vi "main.vi"() -> ()   [LabVIEW 2015]
panel:
  in  "Attenuation":string(combo)
  in  "Level":dbl
  in  "Cmos":string(combo)
  in  "Duty":dbl
  in  "Modulation":string(combo)
  in  "Frequency":dbl
  in  "Range":string(combo)
  in  "Offset":dbl
  in  "Counter":string(combo)
  out "error in":errorcluster
  out "error out":errorcluster
  in  "Function type":string(combo)
  in  "close":bool=TRUE
  out "VISA resource name out":refnum<visa-resource-name>
  in  "open":bool=TRUE
  in  "VISA resource name":refnum<visa-resource-name>
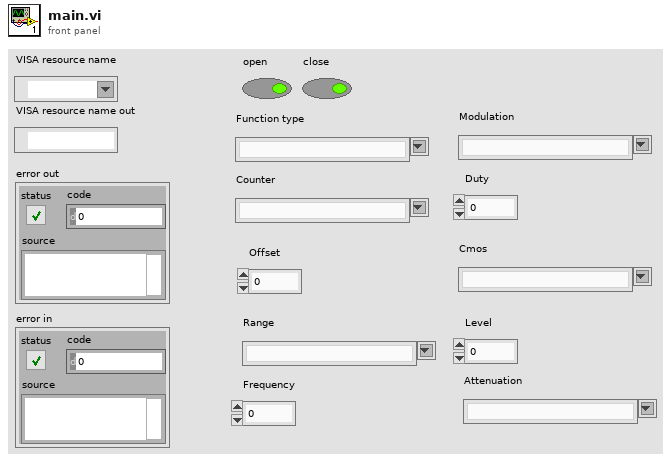
[diagram p1: front panel]
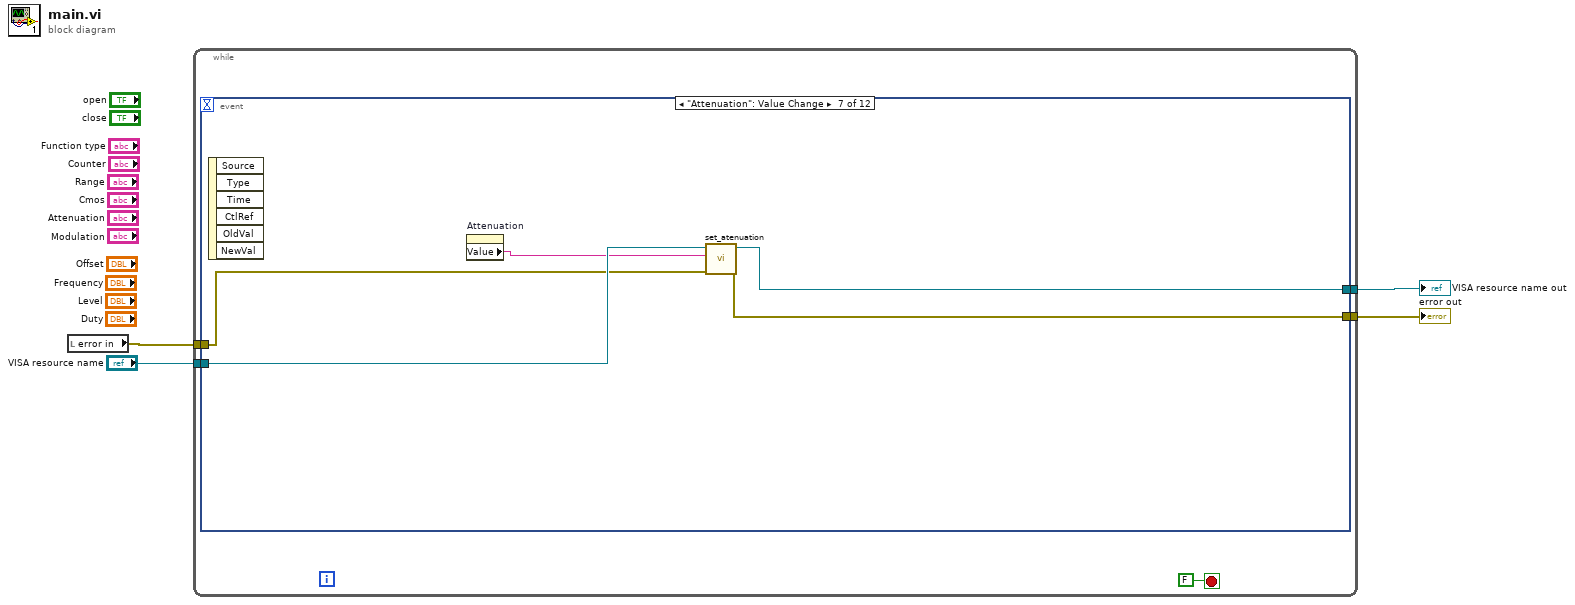
[diagram p0: block diagram]
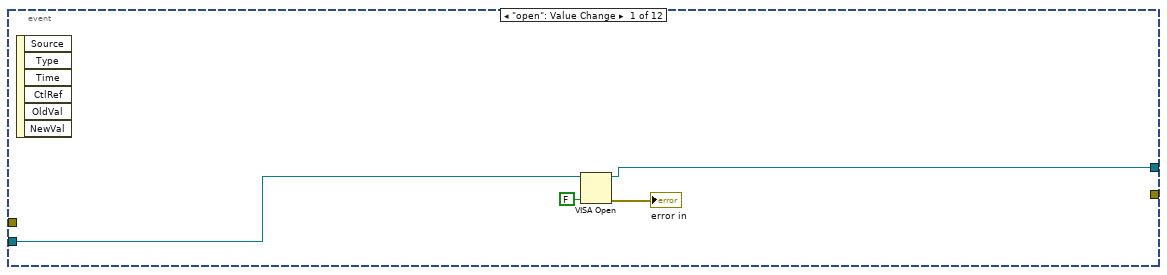
[diagram p2: hidden frame]
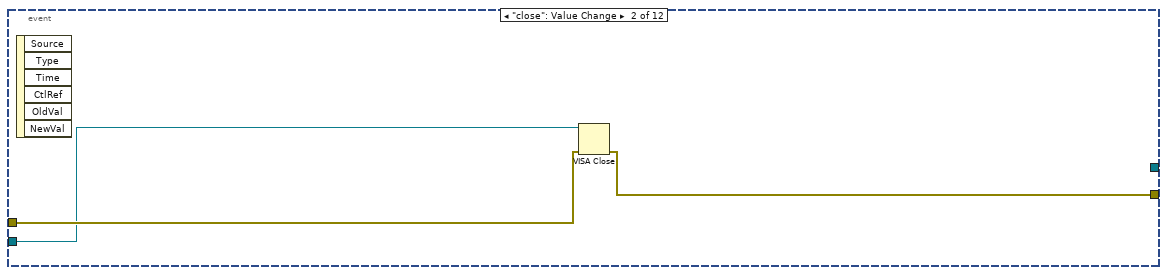
[diagram p3: hidden frame]
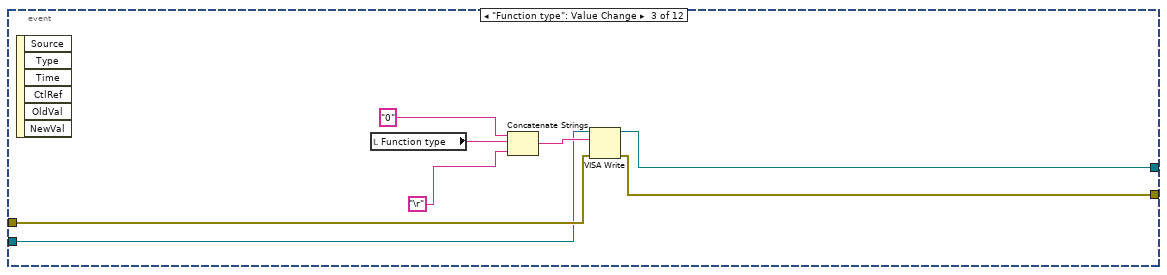
[diagram p4: hidden frame]
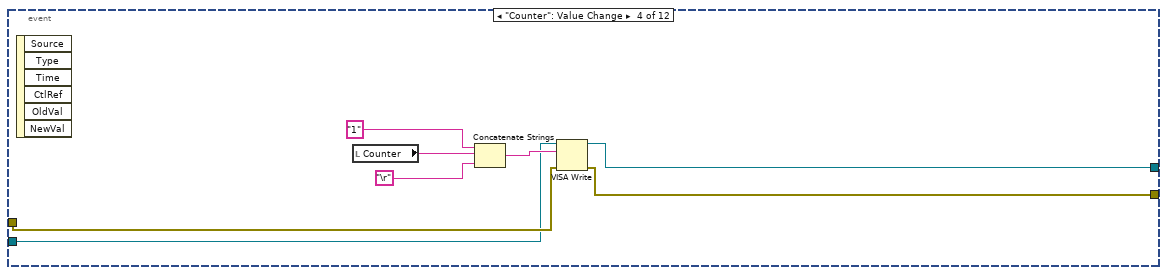
[diagram p5: hidden frame]
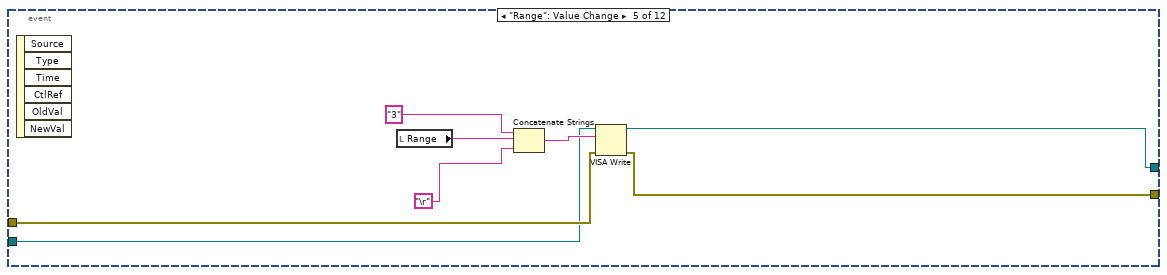
[diagram p6: hidden frame]
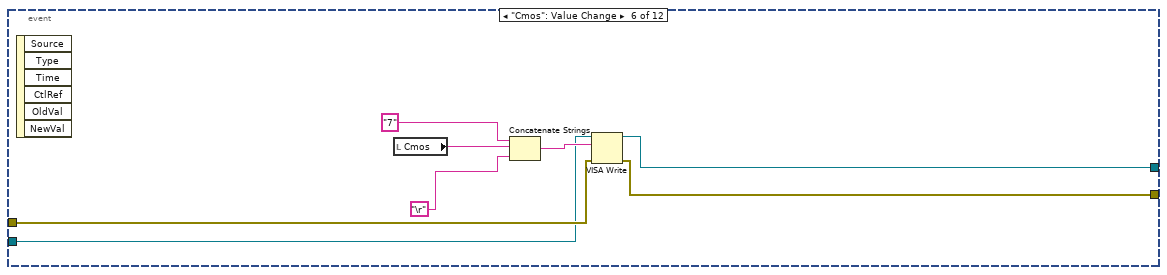
[diagram p7: hidden frame]
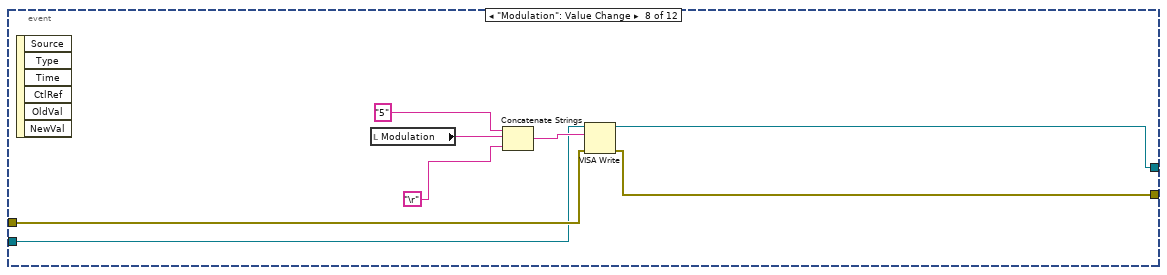
[diagram p8: hidden frame]
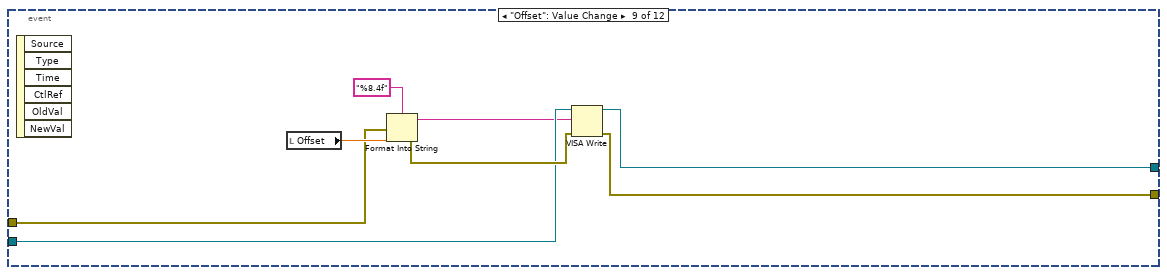
[diagram p9: hidden frame]
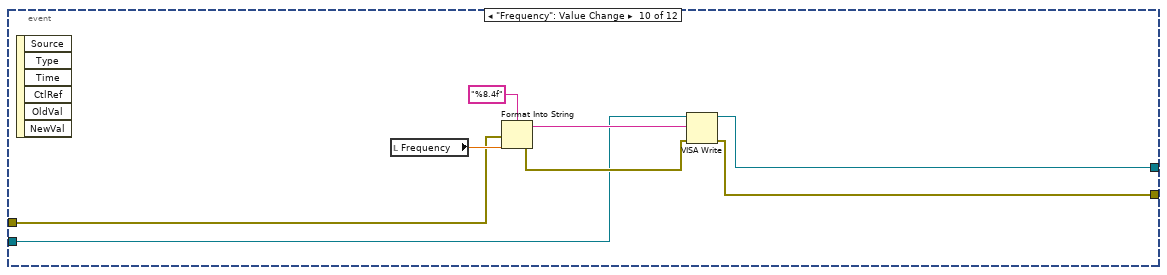
[diagram p10: hidden frame]
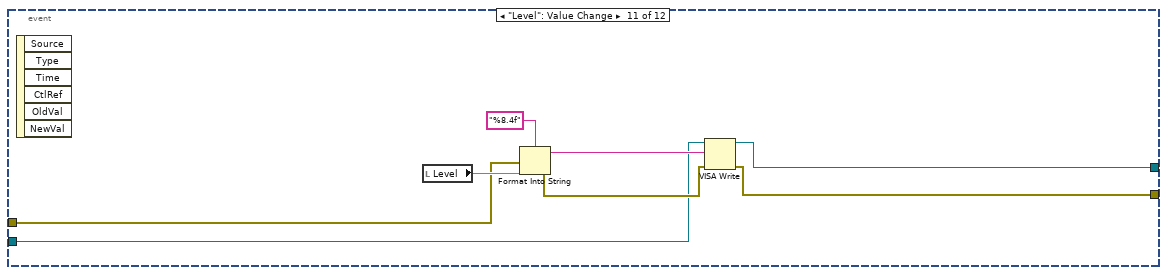
[diagram p11: hidden frame]
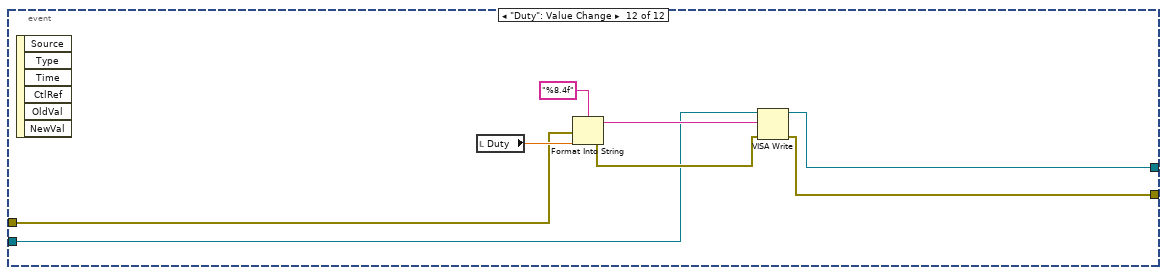
[diagram p12: hidden frame]
diagram:
  n1 = local read "error in"() -> (w4:errorcluster)
  n2 = while {
    tunnel: w4 -> [w8]
    tunnel: [w7] -> w3
    tunnel: "VISA resource name" -> [w6]
    tunnel: [w5] -> w1
    stop <- FALSE ("stop") stop-if-true
    n3 = event shown="[6] \"Attenuation\": Value Change" {
      selector: _ -> [_ _ _ _ _ _ _ _ _ _ _ _]
      dyn-events: _ -> [_ _ _ _ _ _ _ _ _ _ _ _]
      timeout: _ -> [_ _ _ _ _ _ _ _ _ _ _ _]
      tunnel: w8 -> [_ w16 w20 w28 w36 w44 w52 w57 w67 w73 w81 w89]
      tunnel: [_ w15 w19 w27 w33 w42 w50 w54 w65 w70 w79 w86] -> w7
      tunnel: w6 -> [w11 w14 w18 w25 w35 w43 w53 w56 w64 w72 w80 w88]
      tunnel: [w10 _ w17 w26 w34 w41 w51 w55 w62 w71 w78 w87] -> w5
      event "open": Value Change {
        n4 = event-data() -> ()  [unwired: 1 in, 6 out]
        n5 = VISA Open(duplicate session (F)=FALSE, VISA resource name=w11) -> (VISA resource name=w10:refnum<visa-resource-name>, error out=→"error in":errorcluster)  [unwired: 3 in]
      }
      event "close": Value Change {
        n6 = event-data() -> ()  [unwired: 1 in, 6 out]
        n7 = VISA Close(VISA resource name=w14, error in (no error)=w16) -> (error out=w15:errorcluster)
      }
      event "Function type": Value Change {
        n8 = event-data() -> ()  [unwired: 1 in, 6 out]
        n9 = local read "Function type"() -> (w24:string)
        n10 = Concatenate Strings("0" ("string"), w24, "\r") -> (w22:string)
        n11 = VISA Write(VISA resource name=w18, write buffer=w22, error in (no error)=w20) -> (VISA resource name out=w17:refnum<visa-resource-name>, error out=w19:errorcluster)  [unwired: 1 out]
      }
      event "Counter": Value Change {
        n12 = event-data() -> ()  [unwired: 1 in, 6 out]
        n13 = local read "Counter"() -> (w29:string)
        n14 = Concatenate Strings("1" ("string"), w29, "\r") -> (w31:string)
        n15 = VISA Write(VISA resource name=w25, write buffer=w31, error in (no error)=w28) -> (VISA resource name out=w26:refnum<visa-resource-name>, error out=w27:errorcluster)  [unwired: 1 out]
      }
      event "Range": Value Change {
        n16 = event-data() -> ()  [unwired: 1 in, 6 out]
        n17 = local read "Range"() -> (w37:string)
        n18 = Concatenate Strings("3" ("string"), w37, "\r") -> (w39:string)
        n19 = VISA Write(VISA resource name=w35, write buffer=w39, error in (no error)=w36) -> (VISA resource name out=w34:refnum<visa-resource-name>, error out=w33:errorcluster)  [unwired: 1 out]
      }
      event "Cmos": Value Change {
        n20 = event-data() -> ()  [unwired: 1 in, 6 out]
        n21 = local read "Cmos"() -> (w45:string)
        n22 = Concatenate Strings("7" ("string"), w45, "\r") -> (w47:string)
        n23 = VISA Write(VISA resource name=w43, write buffer=w47, error in (no error)=w44) -> (VISA resource name out=w41:refnum<visa-resource-name>, error out=w42:errorcluster)  [unwired: 1 out]
      }
      event "Attenuation": Value Change {
        n24 = event-data() -> ()  [unwired: 1 in, 6 out]
        n25 = property on="Attenuation" class="CmbBox"() -> ("Value"=w49:string)  [unwired: 2 in, 2 out]
        n26 = call "set_atenuation.vi"("error in (no error)"=w52, "Value"=w49, "VISA Refnum in"=w53) -> ("error out"=w50:errorcluster, "VISA Refnum out"=w51:refnum<visa-resource-name>)  [unwired: 7 in]
      }
      event "Modulation": Value Change {
        n27 = event-data() -> ()  [unwired: 1 in, 6 out]
        n28 = local read "Modulation"() -> (w58:string)
        n29 = Concatenate Strings("5" ("string"), w58, "\r") -> (w60:string)
        n30 = VISA Write(VISA resource name=w56, write buffer=w60, error in (no error)=w57) -> (VISA resource name out=w55:refnum<visa-resource-name>, error out=w54:errorcluster)  [unwired: 1 out]
      }
      event "Offset": Value Change {
        n31 = event-data() -> ()  [unwired: 1 in, 6 out]
        n32 = local read "Offset"() -> (w69:dbl)
        n33 = Format Into String(format string="%8.4f", error in=w67, w69) -> (resulting string=w63:string, error out=w66:errorcluster)  [unwired: 1 in]
        n34 = VISA Write(VISA resource name=w64, write buffer=w63, error in (no error)=w66) -> (VISA resource name out=w62:refnum<visa-resource-name>, error out=w65:errorcluster)  [unwired: 1 out]
      }
      event "Frequency": Value Change {
        n35 = event-data() -> ()  [unwired: 1 in, 6 out]
        n36 = local read "Frequency"() -> (w77:dbl)
        n37 = Format Into String(format string="%8.4f", error in=w73, w77) -> (resulting string=w74:string, error out=w75:errorcluster)  [unwired: 1 in]
        n38 = VISA Write(VISA resource name=w72, write buffer=w74, error in (no error)=w75) -> (VISA resource name out=w71:refnum<visa-resource-name>, error out=w70:errorcluster)  [unwired: 1 out]
      }
      event "Level": Value Change {
        n39 = event-data() -> ()  [unwired: 1 in, 6 out]
        n40 = local read "Level"() -> (w85:dbl)
        n41 = Format Into String(format string="%8.4f", error in=w81, w85) -> (resulting string=w82:string, error out=w83:errorcluster)  [unwired: 1 in]
        n42 = VISA Write(VISA resource name=w80, write buffer=w82, error in (no error)=w83) -> (VISA resource name out=w78:refnum<visa-resource-name>, error out=w79:errorcluster)  [unwired: 1 out]
      }
      event "Duty": Value Change {
        n43 = event-data() -> ()  [unwired: 1 in, 6 out]
        n44 = local read "Duty"() -> (w93:dbl)
        n45 = Format Into String(format string="%8.4f", error in=w89, w93) -> (resulting string=w90:string, error out=w91:errorcluster)  [unwired: 1 in]
        n46 = VISA Write(VISA resource name=w88, write buffer=w90, error in (no error)=w91) -> (VISA resource name out=w87:refnum<visa-resource-name>, error out=w86:errorcluster)  [unwired: 1 out]
      }
    }
  }
  "error out" <- w3
  "VISA resource name out" <- w1
